vi "WriteConsiderCorrections.vi"(8 "error in":errorcluster, 9 "Consider SC":bool, 10 "Consider OC":bool, 11 "HP4284A.lvclass in":refnum<class "HP4284A.lvclass">) -> (0 "error out":errorcluster, 3 "HP4284A.lvclass  out":refnum<class "HP4284A.lvclass">)   [LabVIEW 2018, in "HP4284A.lvclass"]
uses:
  HP4284A.lvclass
  HP4284A.lvclass/HP4284A.ctl
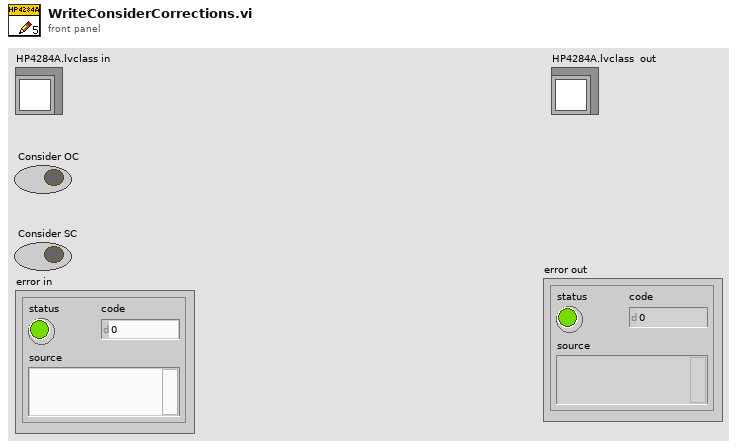
[diagram p1: front panel]
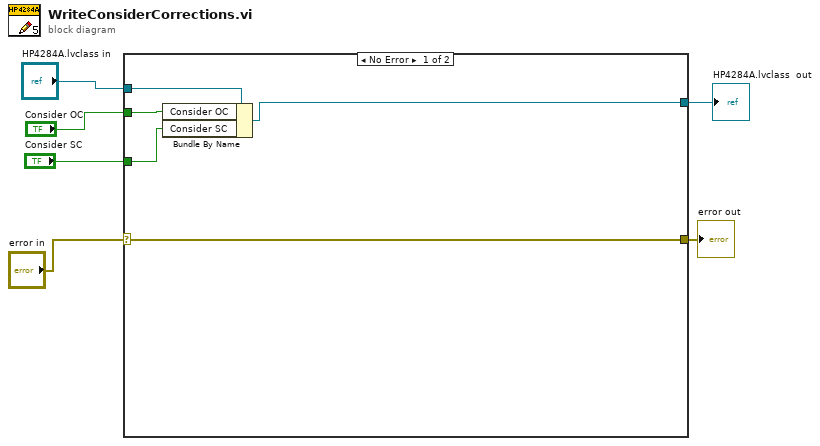
[diagram p0: block diagram]
diagram:
  n1 = case shown="No Error" "error in" {
    selector: "error in" -> [w8 w13]
    tunnel: "HP4284A.lvclass in" -> [w11 w12]
    tunnel: "Consider OC" -> [w10 _]
    tunnel: [w9 w12] -> w4
    tunnel: [w8 w13] -> w2
    tunnel: "Consider SC" -> [w7 _]
    frame No Error {
      n2 = Bundle By Name(cluster=w11, "Consider OC"=w10, "Consider SC"=w7) -> (w9:refnum<class "HP4284A.lvclass">)
    }
    frame Error {
    }
  }
  "HP4284A.lvclass  out" <- w4
  "error out" <- w2
